vi "port detector.vi"(1 "IO":T2) -> (0 "port":T1)   [LabVIEW 2019, in "my FPGA lib.lvlib" / "DIO.lvclass"]
uses:
  DIO.lvclass
  DIO enum.ctl
  port.ctl
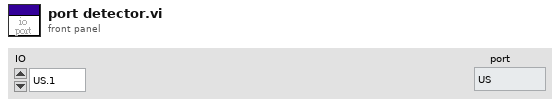
[diagram p1: front panel]
types:
  T1 = typedef "my FPGA lib.lvlib/DIO.lvclass/port.ctl" = enum16{"US", "C.", "B."}
  T2 = typedef "my FPGA lib.lvlib/DIO.lvclass/DIO enum.ctl" = enum16{"US.1", "US.2", "US.3", "US.4", "C.0", "C.1", "C.2", "C.3", "C.4", "C.5", "C.6", "C.7", "B.14", "B.15"}
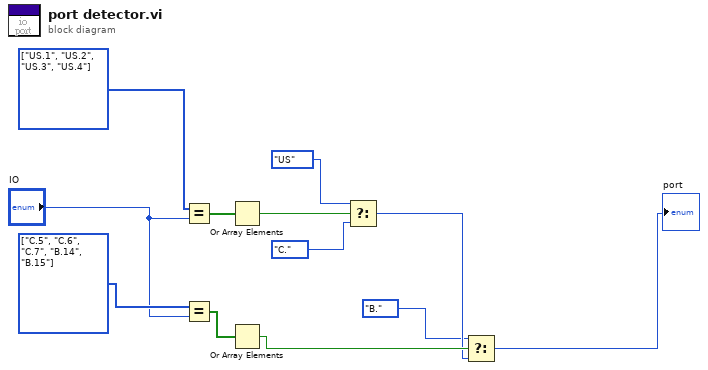
[diagram p0: block diagram]
diagram:
  w7 = T2[] [enum."C.5", enum."C.6", enum."C.7", enum."B.14", enum."B.15"] items=["US.1", "US.2", "US.3", "US.4", "C.0", "C.1", "C.2", "C.3", "C.4", "C.5", "C.6", "C.7", "B.14", "B.15"] ("Array")
  w12 = T2[] [enum."US.1", enum."US.2", enum."US.3", enum."US.4"] items=["US.1", "US.2", "US.3", "US.4", "C.0", "C.1", "C.2", "C.3", "C.4", "C.5", "C.6", "C.7", "B.14", "B.15"] ("Array")
  n1 = Equal?(x=w12, y="IO") -> (x = y?=w11:bool[])
  n2 = Equal?(x=w7, y="IO") -> (x = y?=w5:bool[])
  n3 = Or Array Elements(Boolean array=w11) -> (logical OR=w10:bool)
  n4 = Or Array Elements(Boolean array=w5) -> (logical OR=w4:bool)
  n5 = Select(t=port."US" ("Enum"), s=w10, f=port."C." ("Enum")) -> (s? t:f=w3:T1)
  n6 = Select(t=port."B.", s=w4, f=w3) -> (s? t:f=→"port":T1)
